vi "Decoding_morse.vi"() -> ()   [LabVIEW 2022 SP3]
uses:
  <vilib>/measure/matone.llb/Extract Multiple Tone Information N Chan.vi
  <vilib>/measure/NI_MAPro.lvlib
panel:
  out "Binary detected code":dbl[](array[numeric])
  in  "Jump to analysis":bool=TRUE
  out "Amplitude out":dbl[](array[numeric])
  out "Freq out":dbl[](array[numeric])
  in  "amplit":dbl=1e-05
  in  "high freq":dbl=4800.0
  in  "low freq":dbl=3000.0
  out "error analysis":errorcluster
  in  "Stop analysis":bool
  out "error out listening":errorcluster caption="error out"
  in  "Stop listening":bool
  in  "Sample rate (Hz)":dbl=10000.0
  in  "Duration (s)":dbl=1.0
  out "Input sound":dynamicdata(graph)
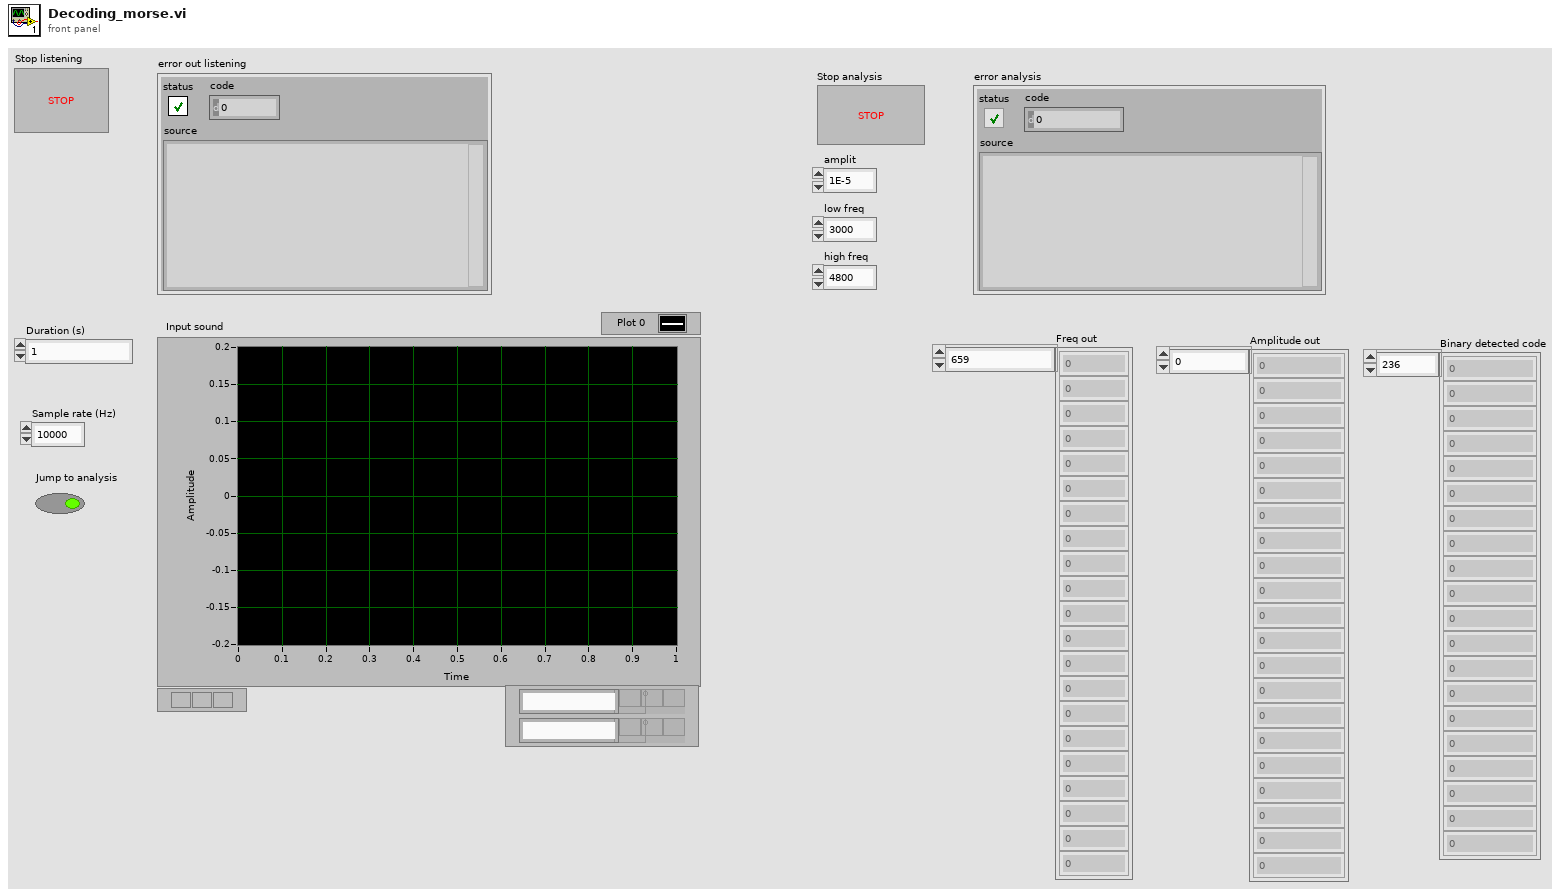
[diagram p1: front panel]
types:
  T1 = cluster{"multiple tone information":cluster{"detected frequency":dbl, "detected amplitude":dbl, "detected phase (deg)":dbl}[]}[]
  T2 = cluster{"multiple tone information":cluster{"detected frequency":dbl, "detected amplitude":dbl, "detected phase (deg)":dbl}[]}
  T3 = cluster{"detected frequency":dbl, "detected amplitude":dbl, "detected phase (deg)":dbl}[]
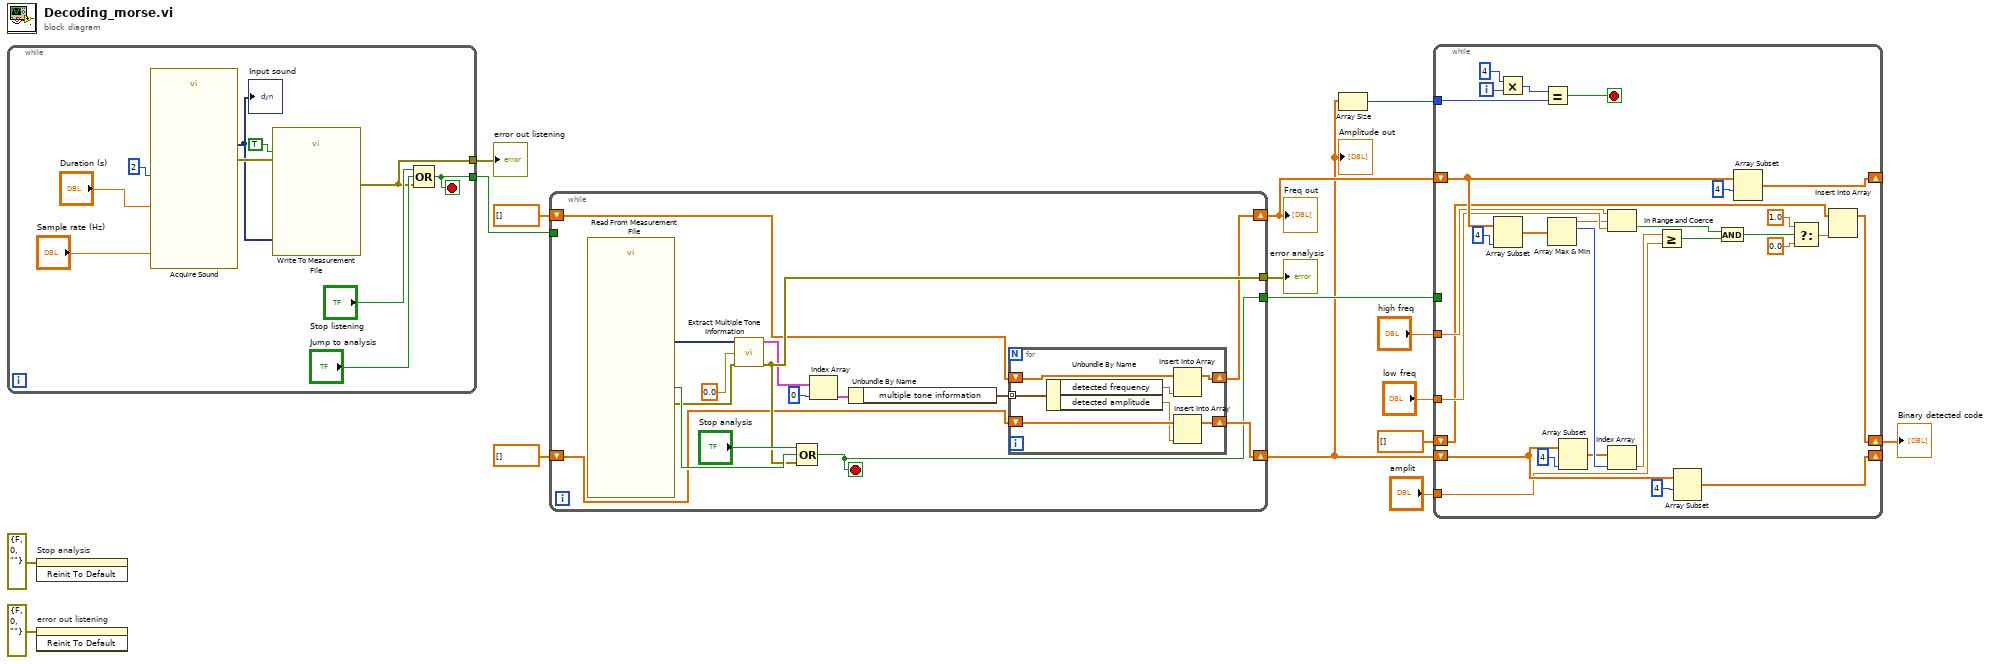
[diagram p0: block diagram]
diagram:
  n1 = while {
    tunnel: [w19] -> w16
    tunnel: [w18] -> w13
    stop <- w18 stop-if-true
    n2 = call "Acquire Sound"("Duration (s)"="Duration (s)", "Sample rate (Hz)"="Sample rate (Hz)", "#Channels"=2) -> ("Data"=w22:dynamicdata, "error out"=w23:errorcluster)  [unwired: 15 in]
    "Input sound" <- w22
    n3 = call "Write To Measurement File"("Signals"=w22, "Enable"=TRUE, "error in (no error)"=w23) -> ("error out"=w19:errorcluster)  [unwired: 14 in, 2 out]
    n4 = Compound Arithmetic op=OR("Stop listening", "Jump to analysis", w19) -> (w18:bool)
  }
  "error out listening" <- w16
  n5 = invoke on="Stop analysis" class="Bool" method="Reinit To Default"(error in=errorcluster {"status"=FALSE, "code"=0, "source"=""} ("error in (no error)")) -> ()  [unwired: 2 in, 3 out]
  n6 = invoke on="error out listening" class="Clust (strict)" method="Reinit To Default"(error in=errorcluster {"status"=FALSE, "code"=0, "source"=""} ("error in (no error)")) -> ()  [unwired: 2 in, 3 out]
  n7 = while {
    tunnel: [w37] -> w12
    shift-right: [w34] -> w2
    shift-left: dbl[] [] ("Amplitude") -> [w35]
    shift-right: [w33] -> w5
    shift-left: dbl[] [] ("Frequency") -> [w36]
    tunnel: w13 -> [_]
    tunnel: [w27] -> w9
    stop <- w27 stop-if-true
    n8 = call "Read From Measurement File"() -> ("error out"=w38:errorcluster, "Signals"=w39:dynamicdata, "EOF?"=w40:bool)  [unwired: 6 in, 3 out]
    n9 = call-poly <vilib>:"Extract Multiple Tone Information.vi"("time signals in"=w39, "threshold"=0.0, "error in (no error)"=w38) -> ("multiple tone information"=w29:T1, "error out"=w37:errorcluster)  [unwired: 10 in, 1 out]
    n10 = Compound Arithmetic op=OR("Stop analysis", w40, w37) -> (w27:bool)
    n11 = Index Array(array=w29, index=0) -> (element=w30:T2)
    n12 = Unbundle By Name(w30) -> ("multiple tone information"=w31:T3)
    n13 = for {
      tunnel: w31 -> [w44] mode=indexing
      shift-right: [w47] -> w33
      shift-left: w36 -> [w48]
      shift-right: [w45] -> w34
      shift-left: w35 -> [w46]
      n14 = Unbundle By Name(w44) -> ("detected frequency"=w43:dbl, "detected amplitude"=w42:dbl)
      n15 = Insert Into Array(array=w48, new element=w43) -> (w47:dbl[])  [unwired: 1 in]
      n16 = Insert Into Array(array=w46, new element=w42) -> (w45:dbl[])  [unwired: 1 in]
    }
  }
  "error analysis" <- w12
  "Freq out" <- w5
  "Amplitude out" <- w2
  n17 = Array Size(array=w2) -> (size(s)=w1:i32)
  n18 = while {
    tunnel: w9 -> [_]
    tunnel: "high freq" -> [w71]
    tunnel: "low freq" -> [w70]
    tunnel: "amplit" -> [w65]
    shift-right: [w68] -> _
    shift-left: w2 -> [w75]
    shift-right: [w74] -> _
    shift-left: w5 -> [w73]
    shift-right: [w58] -> w3
    shift-left: dbl[] [] ("Amplitude") -> [w59]
    tunnel: w1 -> [w56]
    i -> [w51]
    stop <- w55 stop-if-true
    n19 = Array Subset(array=w73, length=4) -> (w72:dbl[])  [unwired: 1 in]
    n20 = Multiply(x=4, y=w51) -> (x*y=w49:i32)
    n21 = Equal?(x=w49, y=w56) -> (x = y?=w55:bool)
    n22 = Array Max & Min(array=w72) -> (max value=w69:dbl, max index (indices)=w67:i32)  [unwired: 2 out]
    n23 = Array Subset(array=w75, length=4) -> (w54:dbl[])  [unwired: 1 in]
    n24 = In Range and Coerce(upper limit=w71, x=w69, lower limit=w70) -> (In Range?=w64:bool)  [unwired: 1 out]
    n25 = Index Array(array=w54, index=w67) -> (element=w66:dbl)
    n26 = Greater Or Equal?(x=w66, y=w65) -> (x >= y?=w63:bool)
    n27 = Array Subset(array=w75, index=4) -> (w68:dbl[])  [unwired: 1 in]
    n28 = And(x=w64, y=w63) -> (x .and. y?=w62:bool)
    n29 = Array Subset(array=w73, index=4 ("x")) -> (w74:dbl[])  [unwired: 1 in]
    n30 = Select(t=1.0, s=w62, f=0.0) -> (s? t:f=w57:dbl)
    n31 = Insert Into Array(array=w59, new element=w57) -> (w58:dbl[])  [unwired: 1 in]
  }
  "Binary detected code" <- w3
